vi "Filter Invalid Plugins.vi"(8 "error in (no error)":errorcluster, 11 "Full Plugin Array":T1[](array[typedef])) -> (0 "error out":errorcluster, 1 "Invalid Plugins":T1[](array[typedef]), 3 "Valid plugins":T1[](array[typedef]))   [LabVIEW 2020, in "RxnRover.lvlib" / "Plugin Manager.lvlib"]
doc: "Filter for valid plugins and sort them into two different plugin.ctl arrays, Valid Plugins which should continute to be loaded and fitlered, and invalid plugins which will be logged and notified to the user. \n\nCreated 5/15/2025 - Labview 2020\nRxnRover"
uses:
  Plugin Manager.lvlib
  Plugin Details.ctl
  Plugin Servers/Controller/Controller Type.ctl
  Plugin Types.ctl
  Config Error.ctl
  Plugin Servers/Controller/Generic Plugin.lvclass
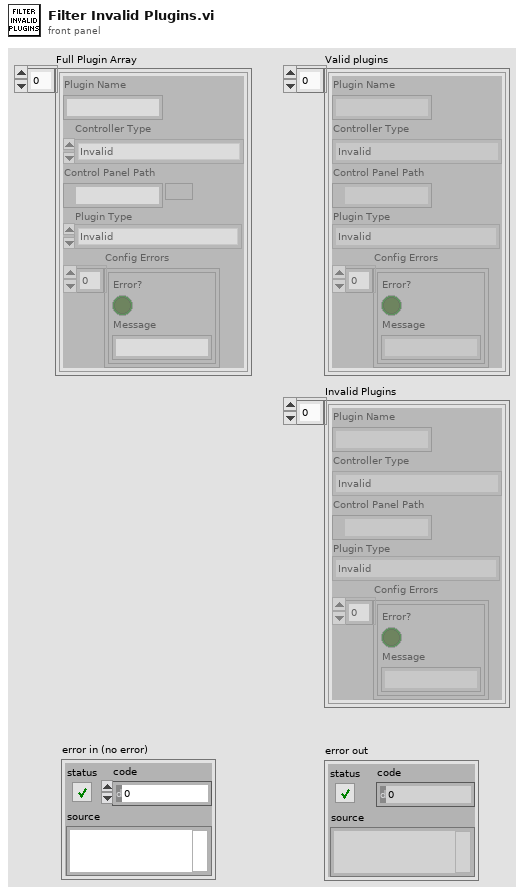
[diagram p1: front panel]
types:
  T1 = typedef "RxnRover.lvlib/Plugin Manager.lvlib/Plugin Details.ctl" = cluster{"Plugin Name":string, "Controller Type":T2, "Control Panel Path":path, "Plugin Type":T3, "Config Errors":T4[]}
  T2 = typedef "RxnRover.lvlib/Generic Plugin.lvclass/Controller Type.ctl" = enum16{"Invalid", "Temperature Controller", "Pump Controller", "Syringe Pump", "Generic Optimizer", "LC Parser", "Passive Hardware"}
  T3 = typedef "RxnRover.lvlib/Plugin Manager.lvlib/Plugin Types.ctl" = enum16{"Invalid", "Optimizer", "Analyzer", "Hardware"}
  T4 = typedef "RxnRover.lvlib/Plugin Manager.lvlib/Config Error.ctl" = cluster{"Error?":bool, "Message":string}
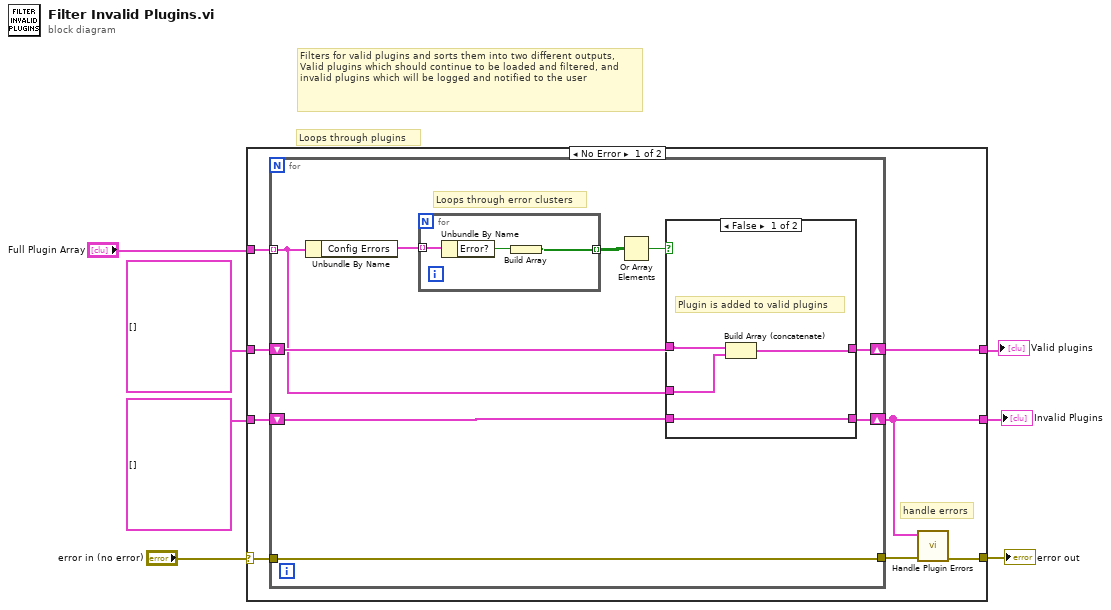
[diagram p0: block diagram]
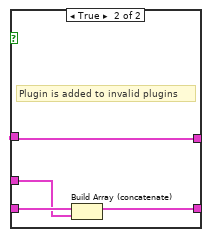
[diagram p2: hidden frame]
diagram:
  # "Loops through plugins"
  # "Filters for valid plugins and sorts them into two different outputs, Valid plugins which should continue to be loaded and filtered, and invalid plugins which will be logged and notified to the user"
  n1 = case shown="No Error" "error in (no error)" {
    selector: "error in (no error)" -> [w11 w36]
    tunnel: "Full Plugin Array" -> [w15 _]
    tunnel: T1[] [] ("Plugin Array") -> [w14 w37]
    tunnel: T1[] [] ("Plugin Array") -> [w13 w38]
    tunnel: [w12 w37] -> w4
    tunnel: [w8 w38] -> w3
    tunnel: [w10 w36] -> w2
    frame No Error {
      # "handle errors"
      n2 = for {
        tunnel: w15 -> [w20] mode=indexing
        tunnel: [w16] -> w9
        shift-right: [w18] -> w12
        shift-left: w14 -> [w21]
        shift-right: [w17] -> w8
        shift-left: w13 -> [w19]
        tunnel: w11 -> [w16]
        # "Loops through error clusters"
        n3 = Unbundle By Name(w20) -> ("Config Errors"=w24:T4[])
        n4 = for {
          tunnel: w24 -> [w35] mode=indexing
          tunnel: [w33] -> w23 mode=indexing
          n5 = Unbundle By Name(w35) -> ("Error?"=w34:bool)
          n6 = Build Array(w34) -> (w33:bool[])
        }
        n7 = Or Array Elements(Boolean array=w23) -> (logical OR=w22:bool)
        n8 = case shown="False" w22 {
          tunnel: w21 -> [w27 w29]
          tunnel: w20 -> [w28 w30]
          tunnel: [w26 w29] -> w18
          tunnel: [w25 w32] -> w17
          tunnel: w19 -> [w25 w31]
          frame False {
            # "Plugin is added to valid plugins"
            n9 = Build Array (concatenate)(w27, w28) -> (w26:T1[])
          }
          frame True {
            # "Plugin is added to invalid plugins"
            n10 = Build Array (concatenate)(w31, w30) -> (w32:T1[])
          }
        }
      }
      n11 = call "Handle Plugin Errors.vi"("error in (no error)"=w9, "Invalid Plugin Array"=w8) -> ("error out"=w10:errorcluster)  [unwired: 9 in]
    }
    frame Error {
    }
  }
  "error out" <- w2
  "Invalid Plugins" <- w3
  "Valid plugins" <- w4
